vi "Pockels Cal_Update single cal section.vi"(10 "New cal section":string[][](array[string])=[["Cal Wavelength", "", "", ""], ["820", "", "", ""], ["Prism 1:", "2039", "", ""], ["Prism 2:", "1953", "", ""], ["Laser power displayed (mW):", "3960", "", ""], ["Pockels bias:", "199", "", ""], ["Zoom:", "12", "", ""], ["Dwell time:", "0.4", "", ""], ["Cal subset indexes", "", "", ""], ["0", "14", "", ""], ["Cal data", "", "", ""], ["Pockels V", "No objective", "Brand new", "Olympus 60X"], ["0", "0", "11", "77"], ["0.1", "2.8", "22", "88"], ["0.2", "9.8", "33", "99"], ["0.3", "21.4", "", ""], ["0.4", "37.1", "", ""], ["0.5", "56.1", "", ""], ["0.6", "77.7", "", ""], ["0.7", "101", "", ""], ["0.8", "125", "", ""], ["0.9", "148", "", ""], ["1", "169", "", ""], ["1.1", "188", "", ""], ["1.2", "204", "", ""], ["1.3", "215", "", ""], ["1.4", "222", "", ""], ["1.5", "225", "", ""], ["1.6", "222", "", ""], ["1.7", "214", "", ""], ["1.8", "202", "", ""], ["1.9", "187", "", ""], ["2", "152", "", ""]], 11 "Loaded cal section":string[][](array[string])=[["Cal Wavelength", "", "", ""], ["820", "", "", ""], ["Prism 1:", "2039", "", ""], ["Prism 2:", "1953", "", ""], ["Laser power displayed (mW):", "3960", "", ""], ["Pockels bias:", "199", "", ""], ["Zoom:", "12", "", ""], ["Dwell time:", "0.4", "", ""], ["Cal subset indexes", "", "", ""], ["0", "14", "", ""], ["Cal data", "", "", ""], ["Pockels V", "No objective", "Olympus 60X", "Olympus 20X"], ["0", "0", "1", "7"], ["0.1", "2.8", "2", "8"], ["0.2", "9.8", "3", "9"], ["0.3", "21.4", "", ""], ["0.4", "37.1", "", ""], ["0.5", "56.1", "", ""], ["0.6", "77.7", "", ""], ["0.7", "101", "", ""], ["0.8", "125", "", ""], ["0.9", "148", "", ""], ["1", "169", "", ""], ["1.1", "188", "", ""], ["1.2", "204", "", ""], ["1.3", "215", "", ""], ["1.4", "222", "", ""], ["1.5", "225", "", ""], ["1.6", "222", "", ""], ["1.7", "214", "", ""], ["1.8", "202", "", ""], ["1.9", "187", "", ""], ["2", "152", "", ""]]) -> (2 "Updated cal section":string[][](array[string]))   [LabVIEW 2017]
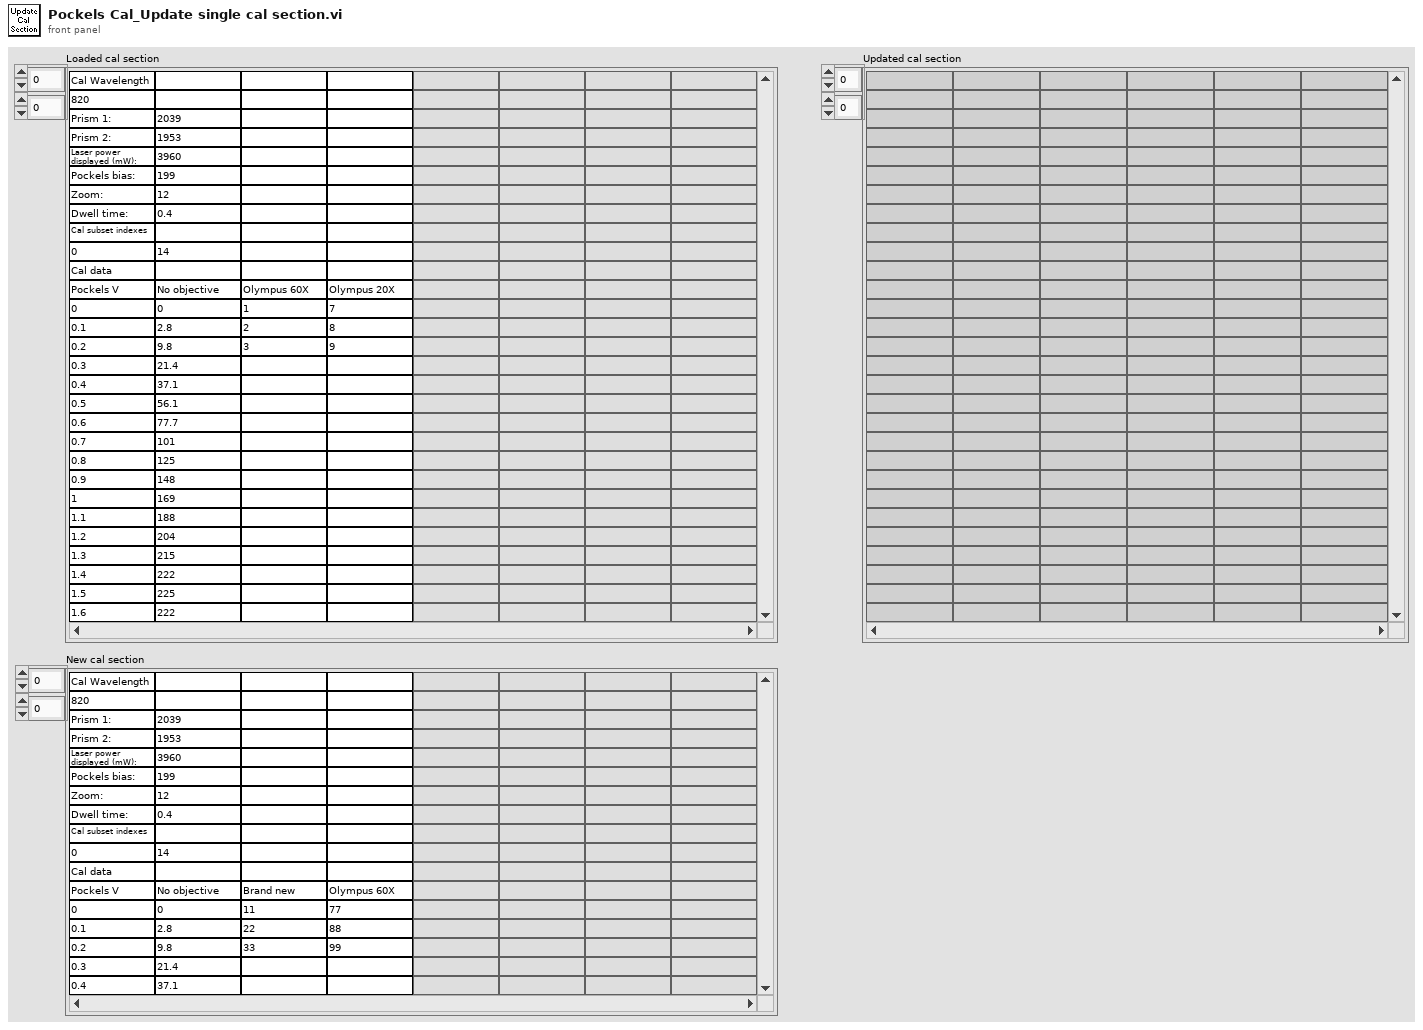
[diagram p1: front panel]
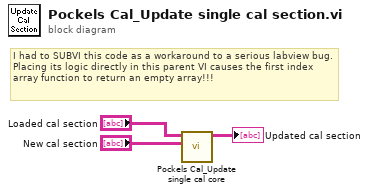
[diagram p0: block diagram]
diagram:
  # "I had to SUBVI this code as a workaround to a serious labview bug. Placing its logic directly in this parent VI causes the first index array function to return an empty array!!!"
  n1 = call "Pockels Cal_Update single cal core.vi"("New cal section"="New cal section", "Loaded cal section"="Loaded cal section") -> ("Updated cal section"=→"Updated cal section":string[][])  [unwired: 9 in]
